vi "PPR_TRAJ_BEGIN.vi"(9 "Initial Gyo Reading":T3 {"SIN" format="%13.4f"; "COS" format="%13.4f"; "VALUE" format="%13.4f"}, 10 "Robot Starting Pose":T1 {"ROTATION"."SIN" format="%13.4f"; "ROTATION"."COS" format="%13.4f"; "ROTATION"."VALUE" format="%13.4f"; "TRANSLATION"."Y" format="%14.3f"; "TRANSLATION"."X" format="%14.3f"}) -> ()   [LabVIEW 2019]
uses:
  PPR_TRAJECTORY_GLOBALS.vi
  <vilib>/Rock Robotics/WPI/ThirdParty/JAS_Junk/TrajLib/TypeDef/TRANSLATION2D.ctl
  <vilib>/Rock Robotics/WPI/ThirdParty/JAS_Junk/TrajLib/Trajectory_Library.lvlib
  <vilib>/Rock Robotics/WPI/ThirdParty/JAS_Junk/TrajLib/TypeDef/ROTATION2D.ctl
  <vilib>/Rock Robotics/WPI/ThirdParty/JAS_Junk/TrajLib/TypeDef/POSE2D.ctl
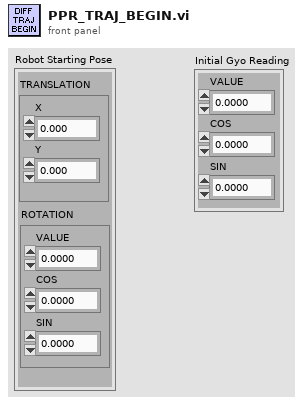
[diagram p1: front panel]
types:
  T1 = typedef "Trajectory_Library.lvlib/POSE2D.ctl" = cluster{"TRANSLATION":T2, "ROTATION":T3}
  T2 = typedef "Trajectory_Library.lvlib/TRANSLATION2D.ctl" = cluster{"X":dbl, "Y":dbl}
  T3 = typedef "Trajectory_Library.lvlib/ROTATION2D.ctl" = cluster{"VALUE":dbl, "COS":dbl, "SIN":dbl}
  T4 = typedef "PathPlanner24.lvlib/PathPlannerTrajectory.ctl" = cluster{"States":T5[]}
  T5 = typedef "PathPlanner24.lvlib/PathPlannerTrajectoryState.ctl" = cluster{"TimeSeconds":dbl, "VelocityMPS":dbl, "AccerationMpsSq":dbl, "HeadingAngularVelRadPerSec":dbl, "PositionMeters":T2, "Heading":T3, "TargetHolonomicRotation":T3, "CurvatureRadPerMeter":dbl, "PathPlannerConstraints":T6, "DeltaPos":dbl}
  T6 = typedef "PathPlanner24.lvlib/PathPlannerPathConstraints.ctl" = cluster{"MaxVelocityMps;":dbl, "MaxAccelerationMpsSq;":dbl, "MaxAngularVelRadPsEc;":dbl, "MaxAngularAccRadPSecSq":dbl, "Exists":bool}
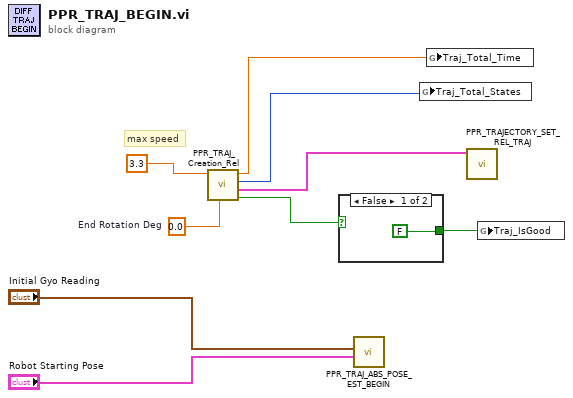
[diagram p0: block diagram]
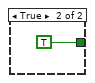
[diagram p2: hidden frame]
diagram:
  w1 = 0.0  # End Rotation Deg
  # "max speed"
  n1 = call "PPR_TRAJ_Creation_Rel.vi"("End Rotation Deg"=w1, "Max Velocity M/S"=3.3 ("Max Velocity Ft/Sec")) -> ("Path\nCreation\nError"=w5:bool, "PathPlannerTrajectory"=w3:T4, "Trajectory State\nCount"=w2:i32, "TotalTImeSecs"=w4:dbl)  [unwired: 6 in]
  n2 = case shown="False" w5 {
    tunnel: [FALSE TRUE] -> w6
    frame False {
    }
    frame True {
    }
  }
  n3 = call "PPR_TRAJ_ABS_POSE_EST_BEGIN.vi"("Initial Pose"="Robot Starting Pose", "Initial Gyro Angle"="Initial Gyo Reading") -> ()  [unwired: 9 in, 1 out]
  n4 = global write "PPR_TRAJECTORY_GLOBALS.vi" "Traj_Total_States"(w2) -> ()
  n5 = global write "PPR_TRAJECTORY_GLOBALS.vi" "Traj_Total_Time"(w4) -> ()
  n6 = call "PPR_TRAJECTORY_SET_REL_TRAJ.vi"("Relative_Trajectory"=w3) -> ()  [unwired: 11 in]
  n7 = global write "PPR_TRAJECTORY_GLOBALS.vi" "Traj_IsGood"(w6) -> ()
